vi "Graphic-Generate Color Map.vi"(0 "User":u32[](array[numeric]), 2 "Map":T1(ring), 5 "Size":i32) -> (4 "Colors":u32[](array[colorbox]))   [LabVIEW 2020]
uses:
  <vilib>/Analysis/1siggen.llb/Ramp Pattern by Samples.vi
  <vilib>/Analysis/NI_AALBase.lvlib
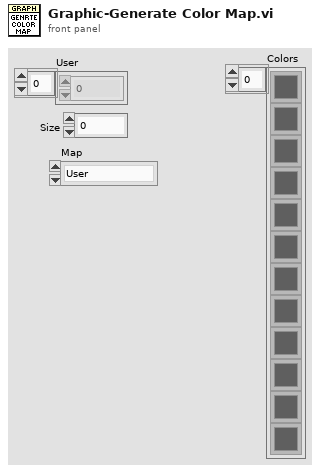
[diagram p1: front panel]
types:
  T1 = enum16{"User", "Prism", "Kelly", "Dark2", "Sequential", "Hue"}
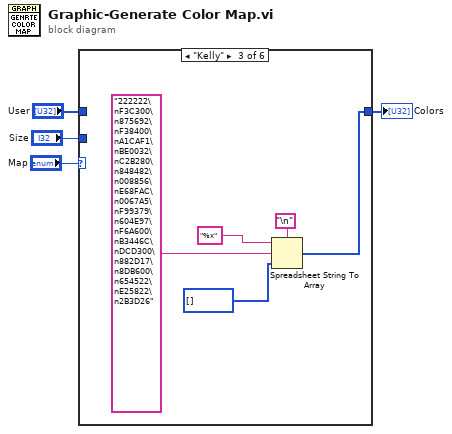
[diagram p0: block diagram]
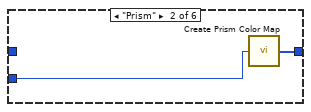
[diagram p3: hidden frame]
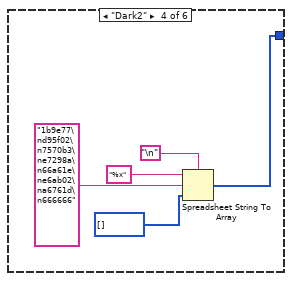
[diagram p4: hidden frame]
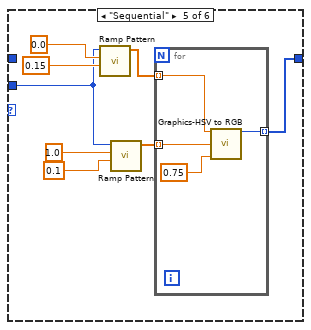
[diagram p5: hidden frame]
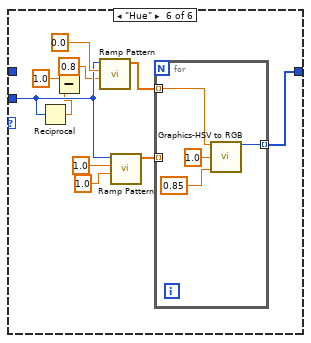
[diagram p6: hidden frame]
diagram:
  n1 = case shown="\"Kelly\"" "Map" {
    tunnel: "User" -> [w5 _ _ _ _ _]
    tunnel: [w5 w7 w8 w14 w25 w39] -> w4
    tunnel: "Size" -> [_ w6 _ _ w20 w32]
    frame "User", Default {
    }
    frame "Prism" {
      n2 = call "Create Prism Color Map.vi"("Size"=w6) -> ("Colors"=w7:u32[])
    }
    frame "Kelly" {
      n3 = Spreadsheet String To Array(delimiter (Tab)="\n", format string="%x", spreadsheet string="222222\nF3C300\n875692\nF38400\nA1CAF1\nBE0032\nC2B280\n848482\n008856\nE68FAC\n0067A5\nF99379\n604E97\nF6A600\nB3446C\nDCD300\n882D17\n8DB600\n654522\nE25822\n2B3D26", array type (2D Dbl)=u32[] []) -> (array=w8:u32[])
    }
    frame "Dark2" {
      n4 = Spreadsheet String To Array(delimiter (Tab)="\n", format string="%x", spreadsheet string="1b9e77\nd95f02\n7570b3\ne7298a\n66a61e\ne6ab02\na6761d\n666666", array type (2D Dbl)=u32[] []) -> (array=w14:u32[])
    }
    frame "Sequential" {
      n5 = call-poly <vilib>:"Ramp Pattern.vi"("start"=0.15 ("x0"), "end"=0.0 ("x0"), "samples"=w20) -> ("Ramp Pattern"=w22:dbl[])  [unwired: 7 in, 1 out]
      n6 = call-poly <vilib>:"Ramp Pattern.vi"("start"=0.1, "end"=1.0, "samples"=w20) -> ("Ramp Pattern"=w21:dbl[])  [unwired: 7 in, 1 out]
      n7 = for {
        tunnel: [w28] -> w25 mode=indexing
        tunnel: w22 -> [w27] mode=indexing
        tunnel: w21 -> [w26] mode=indexing
        n8 = call "Graphics-HSV to RGB.vi"("Hue"=w27, "Saturation"=w26, "Value"=0.75) -> ("Color"=w28:u32)  [unwired: 9 in, 3 out]
      }
    }
    frame "Hue" {
      n9 = Reciprocal(x=w32) -> (1/x=w31:dbl)
      n10 = Subtract(x=1.0 ("x0"), y=w31) -> ()  [unwired: 1 out]
      n11 = call-poly <vilib>:"Ramp Pattern.vi"("start"=0.8, "end"=0.0 ("x0"), "samples"=w32) -> ("Ramp Pattern"=w36:dbl[])  [unwired: 7 in, 1 out]
      n12 = call-poly <vilib>:"Ramp Pattern.vi"("start"=1.0, "end"=1.0, "samples"=w32) -> ("Ramp Pattern"=w35:dbl[])  [unwired: 7 in, 1 out]
      n13 = for {
        tunnel: [w42] -> w39 mode=indexing
        tunnel: w36 -> [w41] mode=indexing
        tunnel: w35 -> [_] mode=indexing
        n14 = call "Graphics-HSV to RGB.vi"("Hue"=w41, "Saturation"=1.0, "Value"=0.85) -> ("Color"=w42:u32)  [unwired: 9 in, 3 out]
      }
    }
  }
  "Colors" <- w4
